vi "Dataset Transaction Id 2 Label.vi"(10 "Dataset Trans Id":T1) -> (2 "Label":string)   [LabVIEW 2009]
uses:
  Dataset Transaction Id.ctl
  Dataset Source.ctl
  Dataset Type.ctl
  Apps/Yes No Button.ctl
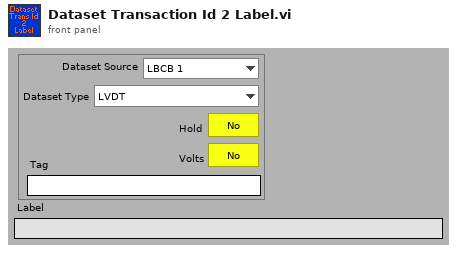
[diagram p1: front panel]
types:
  T1 = typedef "Dataset Transaction Id.ctl" = cluster{"Dataset Source":T2, "Dataset Type":T3, "Hold":T4, "Volts":T4, "Tag":string}
  T2 = typedef "Dataset Source.ctl" = enum16{"LBCB 1", "LBCB 2", "Combined", "External Sensors"}
  T3 = typedef "Dataset Type.ctl" = enum16{"LVDT", "Load Cell", "Actuator Command", "Servo Error", "Displacement Command", "Displacement", "Force"}
  T4 = typedef "Yes No Button.ctl" = bool
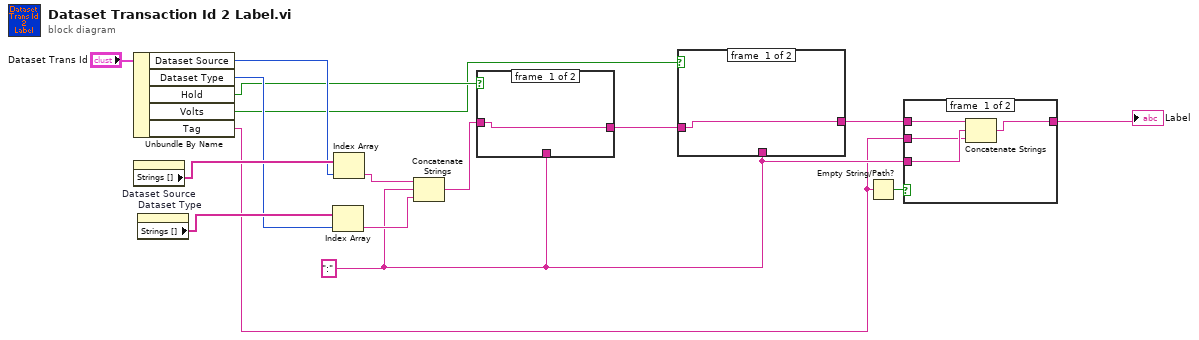
[diagram p0: block diagram]
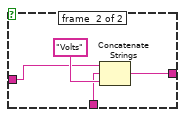
[diagram p3: hidden frame]
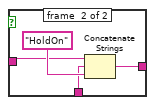
[diagram p4: hidden frame]
diagram:
  w2 = ":"
  n1 = Unbundle By Name("Dataset Trans Id") -> ("Dataset Source"=w14:T2, "Dataset Type"=w12:T3, "Hold"=w9:T4, "Volts"=w8:T4, "Tag"=w1:string)
  n2 = property on="Dataset Source" class="Enum (strict)"() -> ("Strings []"=w15:string[])  [unwired: 2 in, 2 out]
  n3 = property on="Dataset Type" class="Enum (strict)"() -> ("Strings []"=w13:string[])  [unwired: 2 in, 2 out]
  n4 = Index Array(array=w13, index=w12) -> (element=w10:string)
  n5 = Index Array(array=w15, index=w14) -> (element=w11:string)
  n6 = Concatenate Strings(w11, w2, w10) -> (w7:string)
  n7 = case shown="True" w9 {
    tunnel: w7 -> [w17 w19]
    tunnel: w2 -> [_ w20]
    tunnel: [w17 w18] -> w6
    frame #0 {
    }
    frame #1 {
      n8 = Concatenate Strings(w19, w20, "HoldOn" ("string")) -> (w18:string)
    }
  }
  n9 = case shown="True" w8 {
    tunnel: w6 -> [w22 w25]
    tunnel: w2 -> [_ w24]
    tunnel: [w22 w23] -> w4
    frame #0 {
    }
    frame #1 {
      n10 = Concatenate Strings(w25, w24, "Volts" ("string")) -> (w23:string)
    }
  }
  n11 = Empty String/Path?(string/path=w1) -> (empty?=w5:bool)
  n12 = case shown="False" w5 {
    tunnel: w4 -> [w30 w31]
    tunnel: [w29 w31] -> w3
    tunnel: w2 -> [w28 _]
    tunnel: w1 -> [w27 _]
    frame #0 {
      n13 = Concatenate Strings(w30, w28, w27) -> (w29:string)
    }
    frame #1 {
    }
  }
  "Label" <- w3
